vi "DAC Configure.vi"(8 "error in":errorcluster, 11 "DAC Heater Ctrl in":refnum<class "DAC Heater Ctrl.lvclass">) -> (0 "error out":errorcluster, 3 "DAC Heater Ctrl out":refnum<class "DAC Heater Ctrl.lvclass">)   [LabVIEW 2019, in "DAC.lvlib" / "DAC Heater Ctrl.lvclass"]
uses:
  DAC Heater Ctrl.lvclass
  C:/Users/wg/Documents/LV_Projects/TestStand/App/DAC/DAC.lvclass
  DAC.lvclass/DAC.ctl
  DAC Heater Ctrl.lvclass/DAC Heater Ctrl.ctl
  <vilib>/DAQmx/create/channels.llb/DAQmx Create Channel (AO-Voltage-Basic).vi
  DAC.lvclass
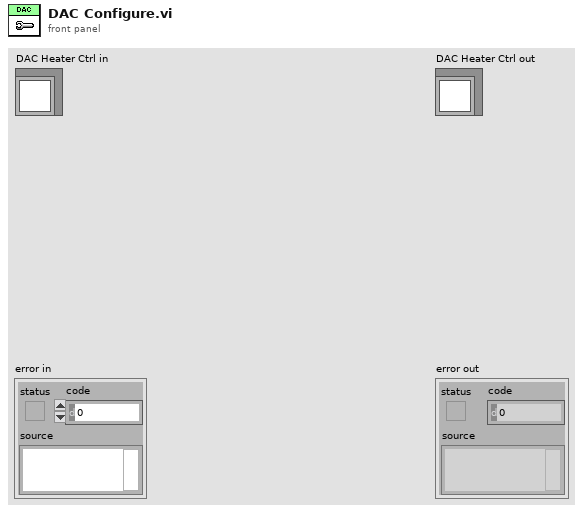
[diagram p1: front panel]
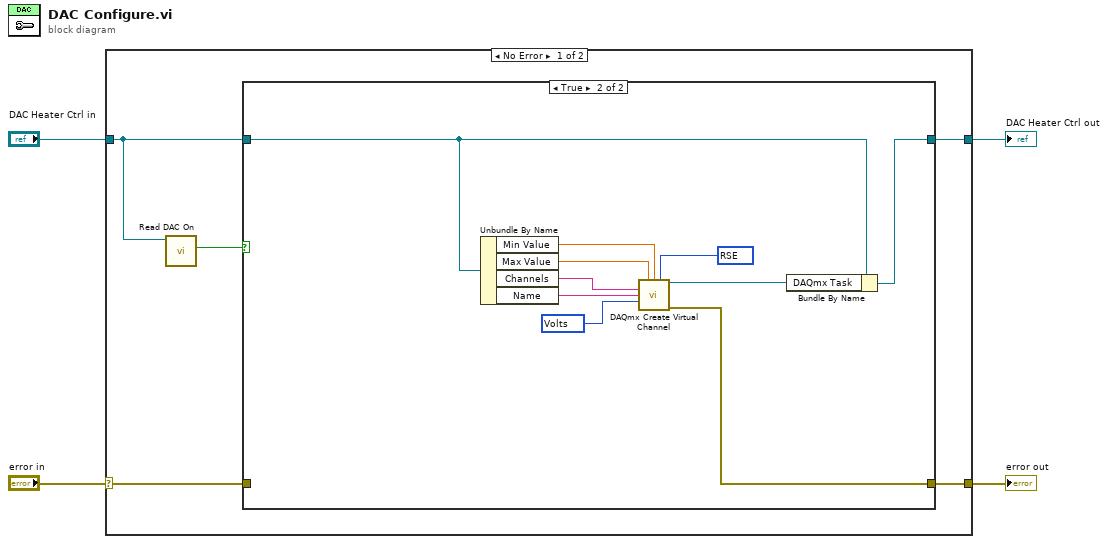
[diagram p0: block diagram]
diagram:
  n1 = case shown="No Error" "error in" {
    selector: "error in" -> [w6 w23]
    tunnel: [w5 w23] -> w4
    tunnel: [w7 w22] -> w3
    tunnel: "DAC Heater Ctrl in" -> [w9 w22]
    frame No Error {
      n2 = call "Read DAC On.vi"("DAC in"=w9) -> ("DAC On"=w8:bool)  [unwired: 8 in, 2 out]
      n3 = case shown="True" w8 {
        tunnel: w9 -> [w11 w20]
        tunnel: [w11 w19] -> w7
        tunnel: w6 -> [w10 _]
        tunnel: [w10 w17] -> w5
        frame False {
          # "Temperature measurement is off."
        }
        frame True {
          w14 = 10083 items=["Default"=-1, "RSE"=10083, "NRSE"=10078, "Differential"=10106, "Pseudodifferential"=12529] ("input terminal configuration")
          w15 = 10348 items=["Volts"=10348, "From Custom Scale"=10065] ("units")
          # "Temperature measurement is on."
          n4 = Unbundle By Name(w20) -> ("Min Value"=w12:dbl, "Max Value"=w21:dbl, "Channels"=w16:string, "Name"=w13:string)
          n5 = call-poly <vilib>:"DAQmx Create Virtual Channel.vi"("maximum value"=w21, "minimum value"=w12, "output terminal configuration"=w14, "physical channels"=w16, "name to assign"=w13, "units"=w15) -> ("task out"=w18:refnum<k21>, "error out"=w17:errorcluster)  [unwired: 8 in]
          n6 = Bundle By Name(cluster=w20, "DAQmx Task"=w18) -> (w19:refnum<class "DAC Heater Ctrl.lvclass">)
        }
      }
    }
    frame Error {
    }
  }
  "error out" <- w4
  "DAC Heater Ctrl out" <- w3
